vi "niLvFpga_ReadFifo_NI 9148.vi"(0 "session in":u32, 1 "scalarType":u32, 2 "bitWidth":u32, 5 "Channel":u32, 7 "Empty Array In":u32[](array[numeric]), 9 "Number Of Elements":u32, 11 "error in":errorcluster, 12 "Timeout(ms)":i32=-1) -> (4 "session out":u32, 8 "Data Out":u32[](array[numeric]), 10 "Remaining":u32, 15 "error out":errorcluster)   [LabVIEW 2017]
doc: "Performance related peculiarities:\n\n1. Disable the Call Library Function's \"Generate Wrappers\" feature. This feature is displayed when you add the following labview.ini token, and right click on the Call Library Function node:\nextFuncGenNoWrapperEnabled=True\n\n2. For the Call Library function, enable \"Constant\" for parameters >> session.\n\n3. Remove the error case structure around the Call Library Functions. Chaining the errors between multiple Call Library Functions will suffice."
uses:
  <vilib>/rvi/errors/niLvFpgaWhatHappensToTopLevelVI.ctl
  <vilib>/rvi/interface/common/niFpgaNodeNameForErrorReporting.ctl
  <vilib>/rvi/interface/common/niFpgaWaitOnOcc.vi
  NiFpgaLv.dll
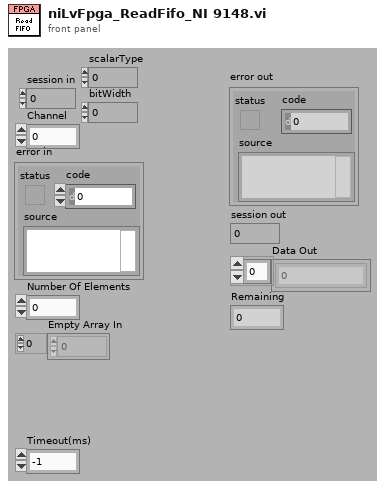
[diagram p1: front panel]
types:
  T1 = typedef "niFpgaNodeNameForErrorReporting.ctl" = enum16{"Open FPGA VI Reference", "Read/Write Control", "Invoke Method: Abort", "Invoke Method: Acknowledge IRQ", "Invoke Method: Download", "Invoke Method: FIFO.Configure", "Invoke Method: FIFO.Read", "Invoke Method: FIFO.Start", "Invoke Method: FIFO.Stop", "Invoke Method: FIFO.Write", "Invoke Method: Reset", "Invoke Method: Run", "Invoke Method: Wait on IRQ", "Close FPGA VI Reference", "Invoke Method: FIFO.Acquire Read Region", "Invoke Method: FIFO.Acquire Write Region"}
  T2 = typedef "niLvFpgaWhatHappensToTopLevelVI.ctl" = enum16{"top level VI scripted behind XNode", "top level VI inlined behind XNode"}
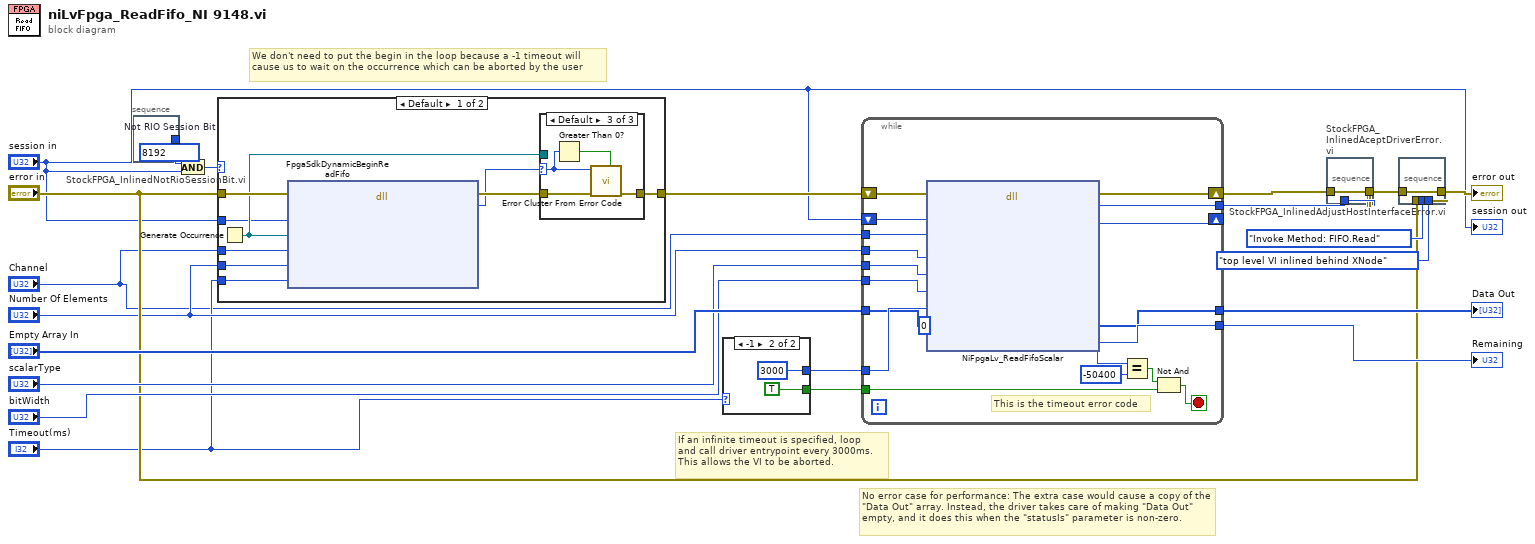
[diagram p0: block diagram]
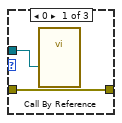
[diagram p4: hidden frame]
diagram:
  # "We don't need to put the begin in the loop because a -1 timeout will cause us to wait on the occurrence which can be aborted by the user"
  # "No error case for performance: The extra case would cause a copy of the \"Data Out\" array. Instead, the driver takes care of making \"Data Out\" empty, and it does this when the \"statusIs\" parameter is non-zero."
  # "If an infinite timeout is specified, loop\nand call driver entrypoint every 3000ms.\nThis allows the VI to be aborted."
  n1 = stacked-sequence "StockFPGA_InlinedNotRioSessionBit.vi" {
    tunnel: [w22] -> w7
    frame #0 {
      w22 = u32 8192  # Not RIO Session Bit
    }
  }
  n2 = And(x=w7, y="session in") -> (x .and. y?=w8:u32)
  n3 = case shown="Default" w8 {
    tunnel: "error in" -> [w30 w39]
    tunnel: [w31 w39] -> w5
    tunnel: "session in" -> [w27 _]
    tunnel: "Channel" -> [w26 _]
    tunnel: "Number Of Elements" -> [w25 _]
    tunnel: "Timeout(ms)" -> [w24 _]
    frame Default {
      n4 = Generate Occurrence() -> (w28:refnum<k4>)
      n5 = dll-call lib="LabVIEW" fn="FpgaSdkDynamicBeginReadFifo"(error in=w30, "session"=w27, "occurrence"=w28, "channel"=w26, "numberOfElements"=w25, "timeout"=w24) -> (error out=w29:errorcluster, "status"=w23:i32)  [unwired: 7 in, 1 out]
      n6 = case shown="Default" w23 {
        selector: w23 -> [_ _ w36]
        tunnel: [w33 w34 w38] -> w31
        tunnel: w28 -> [w32 _ _]
        tunnel: w29 -> [w33 w34 w35]
        frame 0 {
          n7 = call-by-ref "?"("occurrence"=w32) -> ()  [unwired: 16 in, 3 out]
        }
        frame -61167 {
          # "emulation case intentionally ignoring error"
        }
        frame Default {
          n8 = Greater Than 0?(x=w36) -> (x > 0?=w37:bool)
          n9 = call <vilib>:"Error Cluster From Error Code.vi"("is warning? (False)"=w37, "error in (no error)"=w35, "error code (0)"=w36) -> ("error out"=w38:errorcluster)  [unwired: 6 in]
        }
      }
    }
    frame 0 {
    }
  }
  n10 = case shown="-1" "Timeout(ms)" {
    selector: "Timeout(ms)" -> [w40 _]
    tunnel: [w40 3000] -> w20
    tunnel: [_ TRUE] -> w21
    frame Default {
    }
    frame -1 {
    }
  }
  n11 = while {
    tunnel: [w53] -> w11
    tunnel: w21 -> [w57]
    tunnel: w20 -> [w54]
    tunnel: "Number Of Elements" -> [w51]
    tunnel: "Channel" -> [w55]
    tunnel: [w50] -> w19
    shift-right: [w49] -> _
    shift-left: "session in" -> [w56]
    tunnel: "Empty Array In" -> [w48]
    tunnel: [w47] -> w14
    shift-right: [w45] -> w13
    shift-left: w5 -> [w46]
    tunnel: "scalarType" -> [w44]
    tunnel: "bitWidth" -> [w43]
    stop <- w58 stop-if-true
    # "This is the timeout error code"
    n12 = dll-call lib="NiFpgaLv.*" fn="NiFpgaLv_ReadFifoScalar" label="niLvFpgaReadFifo"(error in=w46, "session"=w56, "channel"=w55, "count"=w51, "scalarType"=w44, "bitWidth"=w43, "timeout"=w54, "data"=w48, "remaining"=u32 0 ("elementsRemaining")) -> (error out=w45:errorcluster, "status"=w53:i32, "session"=w49:u32, "data"=w47:u32[], "remaining"=w50:u32)  [unwired: 7 in, 1 out]
    n13 = Equal?(x=w53, y=-50400) -> (x = y?=w59:bool)
    n14 = Not And(1:w57, 2:w59) -> (0:w58:bool)
  }
  "Data Out" <- w14
  "Remaining" <- w19
  n15 = stacked-sequence "StockFPGA_InlinedAceptDriverError.vi" {
    tunnel: w13 -> [w61]
    tunnel: w11 -> [w63]
    tunnel: [w62] -> w12
    frame #0 {
      n16 = case shown="Default" w63 {
        selector: w63 -> [_ w65]
        tunnel: [w64 w67] -> w62
        tunnel: w61 -> [w64 w68]
        frame 0 {
        }
        frame Default {
          n17 = Greater Than 0?(x=w65) -> (x > 0?=w66:bool)
          n18 = call <vilib>:"Error Cluster From Error Code.vi"("is warning? (False)"=w66, "error in (no error)"=w68, "error code (0)"=w65) -> ("error out"=w67:errorcluster)  [unwired: 6 in]
        }
      }
    }
  }
  n19 = stacked-sequence "StockFPGA_InlinedAdjustHostInterfaceError.vi" {
    tunnel: w12 -> [w74]
    tunnel: "error in" -> [w71]
    tunnel: niFpgaNodeNameForErrorReporting."Invoke Method: FIFO.Read" ("node name for error reporting") -> [w69]
    tunnel: niLvFpgaWhatHappensToTopLevelVI."top level VI inlined behind XNode" ("what happens to top level VI") -> [w70]
    tunnel: [w72] -> w16
    frame #0 {
      n20 = Unbundle By Name(w74) -> ("code"=w73:i32)
      n21 = case shown="Default" w73 {
        tunnel: [w75 w80] -> w72
        tunnel: w71 -> [w75 w79]
        tunnel: w70 -> [_ w78]
        tunnel: w69 -> [_ w77]
        tunnel: w74 -> [_ w76]
        frame 0 {
        }
        frame Default {
          n22 = call <vilib>:"niLvFpgaAdjustHostInterfaceError.vi"("error in"=w76, "prior error in"=w79, "node name for error reporting"=w77, "what happens to top level VI"=w78) -> ("error out"=w80:errorcluster)  [unwired: 11 in]
        }
      }
    }
  }
  "error out" <- w16
  "session out" <- "session in"
